vi "IX81 Send Command.vi"(0 "VISA Ref":refnum<visa-resource-name>, 2 "Wait for Reply (T)":bool=TRUE, 7 "Command":string, 11 "Error In":errorcluster) -> (4 "VISA Ref Dup":refnum<visa-resource-name>, 8 "Reply":string, 15 "Error Out":errorcluster)   [LabVIEW 2020]
uses:
  <vilib>/Utility/error.llb/whitespace.ctl
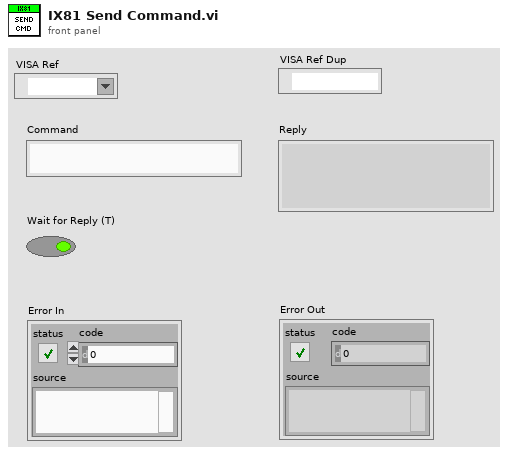
[diagram p1: front panel]
types:
  T1 = typedef "whitespace.ctl" = u16
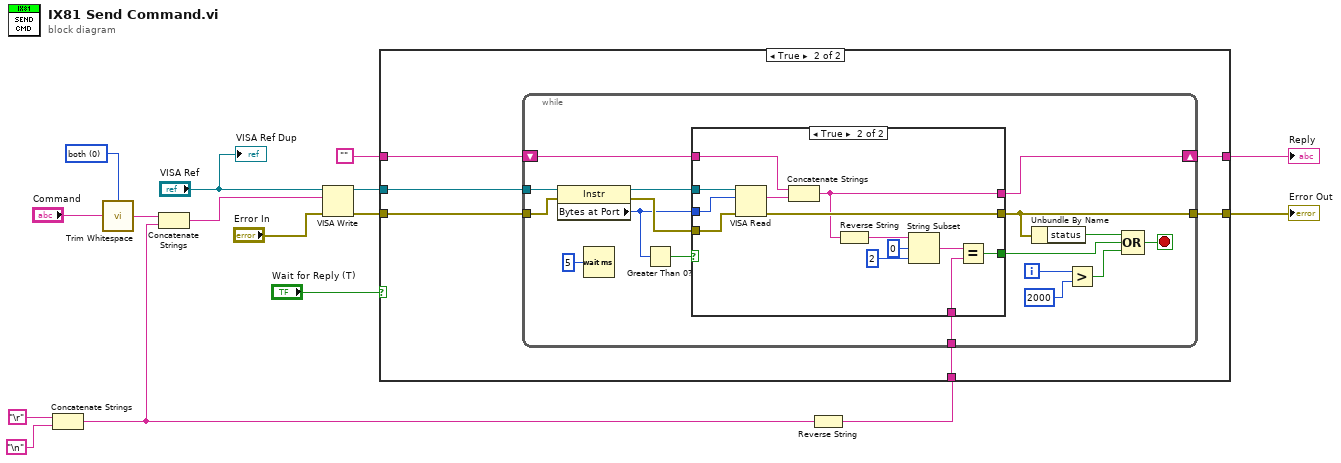
[diagram p0: block diagram]
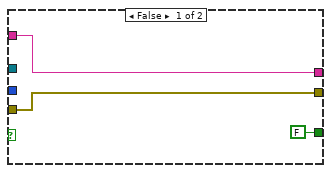
[diagram p3: hidden frame]
diagram:
  w15 = T1 0 items=["both", "start of string", "end of string"] ("location (both)")
  n1 = Concatenate Strings("\r", "\n") -> (w2:string)
  n2 = call <vilib>:"Trim Whitespace.vi"("string"="Command", "location (both)"=w15) -> ("trimmed string"=w14:string)
  n3 = Concatenate Strings(w14, w2) -> (w13:string)
  n4 = VISA Write(VISA resource name="VISA Ref", write buffer=w13, error in (no error)="Error In") -> (VISA resource name out=w12:refnum<visa-resource-name>, error out=w11:errorcluster)  [unwired: 1 out]
  n5 = Reverse String(1:w2) -> (0:w1:string)
  n6 = case shown="True" "Wait for Reply (T)" {
    tunnel: w12 -> [_ w20]
    tunnel: w11 -> [w18 w19]
    tunnel: "" -> [w17 w24]
    tunnel: [w17 w23] -> w5
    tunnel: [w18 w22] -> w7
    tunnel: w1 -> [_ w21]
    frame False {
    }
    frame True {
      n7 = while {
        tunnel: w20 -> [w41]
        tunnel: w19 -> [w40]
        shift-right: [w29] -> w23
        shift-left: w24 -> [w30]
        tunnel: [w26] -> w22
        tunnel: w21 -> [w25]
        i -> [w39]
        stop <- w36 stop-if-true
        n8 = property class="Instr"(reference=w41, error in=w40) -> (reference out=w32:refnum<visa-resource-name>, error out=w33:errorcluster, "Bytes at Port"=w31:u32)
        n9 = Wait (ms)(milliseconds to wait=u32 5) -> ()  [unwired: 1 out]
        n10 = Greater Than 0?(x=w31) -> (x > 0?=w34:bool)
        n11 = case shown="True" w34 {
          tunnel: w33 -> [w43 w56]
          tunnel: w32 -> [_ w57]
          tunnel: w31 -> [_ w55]
          tunnel: w30 -> [w44 w54]
          tunnel: [w44 w51] -> w29
          tunnel: [w43 w52] -> w26
          tunnel: [FALSE w46] -> w27
          tunnel: w25 -> [_ w45]
          frame False {
          }
          frame True {
            n12 = VISA Read(VISA resource name=w57, byte count=w55, error in (no error)=w56) -> (read buffer=w53:string, error out=w52:errorcluster)  [unwired: 2 out]
            n13 = Concatenate Strings(w54, w53) -> (w51:string)
            n14 = Reverse String(1:w51) -> (0:w50:string)
            n15 = String Subset(string=w50, offset (0)=0, length (rest)=2 ("length (rest)")) -> (substring=w47:string)
            n16 = Equal?(x=w47, y=w45) -> (x = y?=w46:bool)
          }
        }
        n17 = Unbundle By Name(w26) -> ("status"=w28:bool)
        n18 = Greater?(x=w39, y=2000) -> (0:w37:bool)
        n19 = Compound Arithmetic op=OR(w28, w27, w37) -> (w36:bool)
      }
    }
  }
  "Reply" <- w5
  "Error Out" <- w7
  "VISA Ref Dup" <- "VISA Ref"
